vi "Vacuum.vi"(8 "error in (no error)":errorcluster, 10 "Vacuum Setting (0000)":i64 min=0 max=1000 step=1 format="%04.0f", 11 "Dispenser in":refnum<class "Dispenser.lvclass">) -> (0 "error out":errorcluster, 3 "Dispenser out":refnum<class "Dispenser.lvclass">)   [LabVIEW 2016, in "Dispenser.lvclass"]
uses:
  Dispenser.lvclass
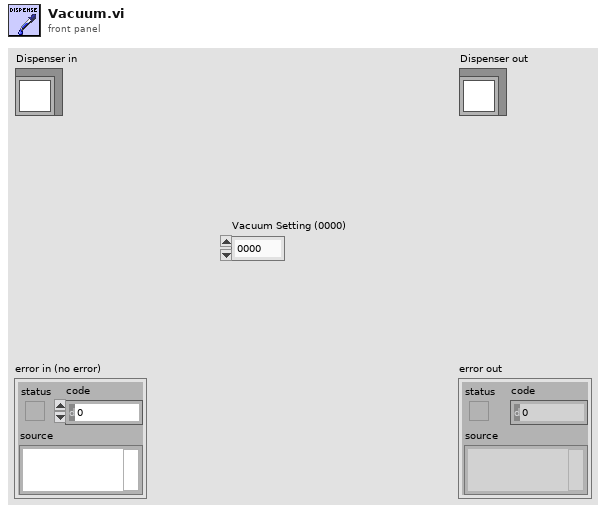
[diagram p1: front panel]
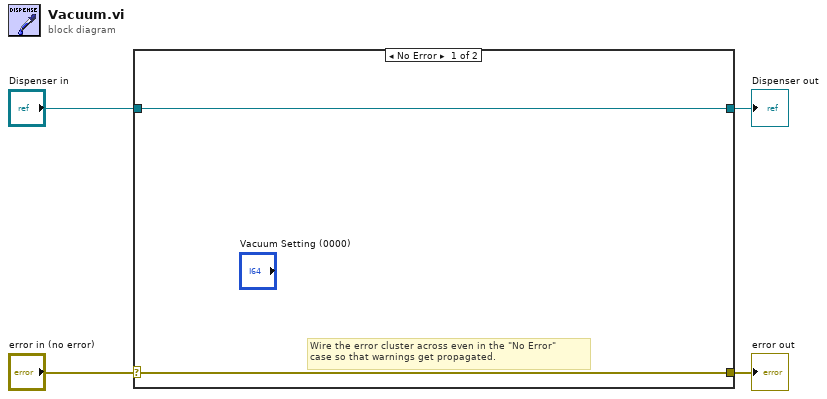
[diagram p0: block diagram]
diagram:
  n1 = case shown="No Error" "error in (no error)" {
    selector: "error in (no error)" -> [w5 w8]
    tunnel: [w5 w8] -> w3
    tunnel: [w6 w7] -> w1
    tunnel: "Dispenser in" -> [w6 w7]
    frame No Error {
      # "Wire the error cluster across even in the \"No Error\"\ncase so that warnings get propagated."
    }
    frame Error {
    }
  }
  "error out" <- w3
  "Dispenser out" <- w1
